vi "Main.vi"(11 "Module Admin":refnum<class "Delacor_lib_QMH_Module Admin.lvclass">) -> ()   [LabVIEW 2019, in "Analysis.lvlib"]
doc: "This template is based off of the Queued Message Handler design pattern and the Queued Message Handler project template that ships with LabVIEW.\n\nThe main difference is that the queue is private to this module and communication between modules is performed via Broadcast and Request events.\n\nRequest events are wrapped in public API methods and are handled in the Event Handling Loop (EHL) of this VI. Any module can register for Broadcast events sent by this module. The EHL generates messages based on user interface actions.\n\nThe Message Handling Loop (MHL) processes messages generated by the EHL, or by other messages. The messages are string values, so new messages can be added easily to the Message Cases case structure in the MHL. Each message cluster can also provide an optional value for Message Data, which is a variant that can be converted to whatever message-specific data is required.\n_____\nBased on Delacor QMH Project Template 4.0.0.47.\n_____\nBased on DQMH Project Template 6.1.0.94."
uses:
  Analysis.lvlib
  <vilib>/Delacor/Delacor QMH/Libraries/Module Admin_class/Delacor_lib_QMH_Module Admin.lvclass
  Module Data--cluster.ctl
  Neo-Laura-LVOOP/Class Library/Fcurve_class/Fcurve.lvclass
  Main UI Shared/Decimation input --cluster.ctl
  Stop Argument--cluster.ctl
  <vilib>/Delacor/Delacor QMH/Libraries/Message Queue_class/Delacor_lib_QMH_Message Queue.lvclass/Delacor_lib_QMH_Message Queue.ctl
  <vilib>/Delacor/Delacor QMH/Libraries/Module Admin_class/Delacor_lib_QMH_Module Admin.lvclass/Delacor_lib_QMH_Module Admin.ctl
  Update analysis parameters Argument--cluster.ctl
  Update analysis parameters (Reply Payload)--cluster.ctl
  Update Savitzky parameters Argument--cluster.ctl
  Update decimation Argument--cluster.ctl
  Update contact parameters Argument--cluster.ctl
  Update Tau delay (ms) Argument--cluster.ctl
  Open Fcurve object Argument--cluster.ctl
  Neo-Laura-LVOOP/SignalViewer/TDMS_DataHandler_class/Fcurve Meta data.ctl
  Open Fcurve object (Reply Payload)--cluster.ctl
  Neo-Laura-LVOOP/Class Library/Fcurve_class/Metadata.ctl
  <vilib>/Utility/miscctls.llb/LVPointTypeDef.ctl
  <vilib>/Delacor/Delacor QMH/Libraries/Message Queue_class/Delacor_lib_QMH_Enqueue Message (Single).vi
  <vilib>/Delacor/Delacor QMH/Libraries/Module Admin_class/Delacor_lib_QMH_Get External Launch.vi
  <vilib>/Utility/error.llb/Error Cluster From Error Code.vi
  <vilib>/ErrorRing/Error Ring.xnode
  <vilib>/Delacor/Delacor QMH/Libraries/Message Queue_class/Delacor_lib_QMH_Message Queue.lvclass
  Settings Editor/Settings Editor.lvlib
  Main UI Shared/MAIN UI Shared.lvlib
  Neo-Laura-LVOOP/SignalViewer/TDMS_DataHandler_class/TDMS_DataHandler.lvclass
panel:
  out "Settings":T1={"Contact"={"Contact stat?"=TRUE, "Contact Spread of dev"=0.0}, "Decimation"={"App"={"Dec"=1, "apply"=FALSE}, "Con"={"Dec"=1, "apply"=FALSE}, "Ret"={"Dec"=1, "apply"=FALSE}}, "Savitzksky-Golay"={"Sidepoints (M)"=20.0, "Filter Order"=5}, "Fcurve Metadata"=[], "Tau Delay (ms)"=0.0, "Fcurve obj"=refnum} {"Savitzksky-Golay"."Filter Order" scale=0.0..10.0; "Savitzksky-Golay"."Sidepoints (M)" scale=0.0..10.0; "Contact"."Contact Spread of dev" format="%#_13g"}
  out "error out":errorcluster
  # "This is a headless module. Show its panel to confirm that the Settings are updated correctly and other debugging tasks. Use the Settings Editor to change the settings for this module."
  # "Contact"
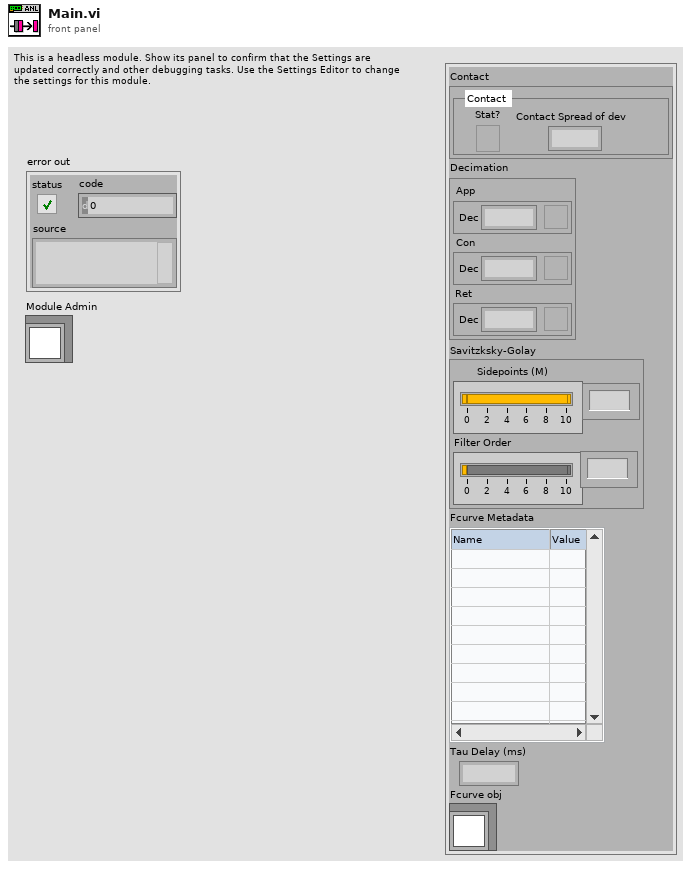
[diagram p1: front panel]
types:
  T1 = typedef "Analysis.lvlib/Module Data--cluster.ctl" = cluster{"Contact":cluster{"Contact stat?":bool, "Contact Spread of dev":dbl}, "Decimation":T2, "Savitzksky-Golay":cluster{"Sidepoints (M)":dbl, "Filter Order":i32}, "Fcurve Metadata":string[][], "Tau Delay (ms)":dbl, "Fcurve obj":refnum<class "Fcurve.lvclass">}
  T2 = typedef "MAIN UI Shared.lvlib/Decimation input --cluster.ctl" = cluster{"App":cluster{"Dec":i32, "apply":bool}, "Con":cluster{"Dec":i32, "apply":bool}, "Ret":cluster{"Dec":i32, "apply":bool}}
  T3 = typedef "Settings Editor.lvlib/Broadcast Events--cluster.ctl" = cluster{"Module Did Init":refnum<user-event>, "Status Updated":refnum<user-event>, "Error Reported":refnum<user-event>, "Module Did Stop":refnum<user-event>, "Update Module Execution Status":refnum<user-event>, "TDMS path settings updated":refnum<user-event>}
  T4 = typedef "Analysis.lvlib/Request Events--cluster.ctl" = cluster{"Stop Module":refnum<user-event>, "Show Panel":refnum<user-event>, "Hide Panel":refnum<user-event>, "Get Module Execution Status":refnum<user-event>, "Show Diagram":refnum<user-event>, "Wakeup Helper Loop":refnum<user-event>, "Change Settings":refnum<user-event>, "Update analysis parameters":refnum<user-event>, "Update Savitzky parameters":refnum<user-event>, "Update decimation":refnum<user-event>, "Update contact parameters":refnum<user-event>, "Update Tau delay (ms)":refnum<user-event>, "Open Fcurve object":refnum<user-event>}
  T5 = enum32{"invalid lock state", "Not Locked", "Locked (No Password)", "Password-protected"}
  T6 = typedef "Analysis.lvlib/Stop Argument--cluster.ctl" = cluster{"Origin":string, "Exit via Stop Module Req?":bool, "Wait for Module to stop?":bool}
  T7 = typedef "Analysis.lvlib/Update analysis parameters Argument--cluster.ctl" = cluster{"Contact":cluster{"Contact stat?":bool, "Contact Spread of dev":dbl}, "Decimation":T2, "Savitzksky-Golay":cluster{"Sidepoints (M)":dbl, "Filter Order":i32}, "Wait Notifier":refnum<notifier>, "wait for reply":bool}
  T8 = typedef "Analysis.lvlib/Update Savitzky parameters Argument--cluster.ctl" = cluster{"Savitzksky-Golay":cluster{"Sidepoints (M)":dbl, "Filter Order":i32}}
  T9 = typedef "Analysis.lvlib/Update decimation Argument--cluster.ctl" = cluster{"Decimation":T2}
  T10 = typedef "Analysis.lvlib/Update contact parameters Argument--cluster.ctl" = cluster{"Contact":cluster{"Contact stat?":bool, "Contact Spread of dev":dbl}}
  T11 = typedef "Analysis.lvlib/Update Tau delay (ms) Argument--cluster.ctl" = cluster{"Tau Delay (ms)":dbl}
  T12 = typedef "Analysis.lvlib/Open Fcurve object Argument--cluster.ctl" = cluster{"Group metadata":T13, "Channel name(s)":string[], "Channel datum out":waveform(dbl)[], "Wait Notifier":refnum<notifier>, "wait for reply":bool}
  T13 = typedef "TDMS_DataHandler.lvclass/Fcurve Meta data.ctl" = cluster{"property names":string[], "property values":variant[]}
  T14 = typedef "LVPointTypeDef.ctl" = cluster{"Horizontal":i16, "Vertical":i16}
  T15 = enum32{"Invalid", "Standard", "Closed", "Hidden", "Minimized", "Maximized"}
  T16 = typedef "Analysis.lvlib/Update analysis parameters (Reply Payload)--cluster.ctl" = cluster{"updated":bool, "error":errorcluster}
  T17 = typedef "Analysis.lvlib/Open Fcurve object (Reply Payload)--cluster.ctl" = cluster{"Fcurve out":cluster{"X":dbl[], "Y":dbl[]}[], "Metadata out":T18, "error":errorcluster}
  T18 = typedef "Fcurve.lvclass/Metadata.ctl" = cluster{"dt (us)":dbl, "Dec Factor":dbl, "Z piezo Sensitivity (nm/V)":dbl, "K (N/m)":dbl, "Sp (V)":dbl, "Contact (ms)":dbl, "Zpos contact":dbl, "Vel_app (nm/s)":dbl, "Vel_ret (nm/s)":dbl, "deltaV (nm)":dbl, "Def_V0 (v)":dbl, "Piezo gain":dbl, "invOLS (nm/V)":dbl}
  T19 = cluster{"Contact stat?":bool, "Contact Spread of dev":dbl}
  T20 = cluster{"Sidepoints (M)":dbl, "Filter Order":i32}
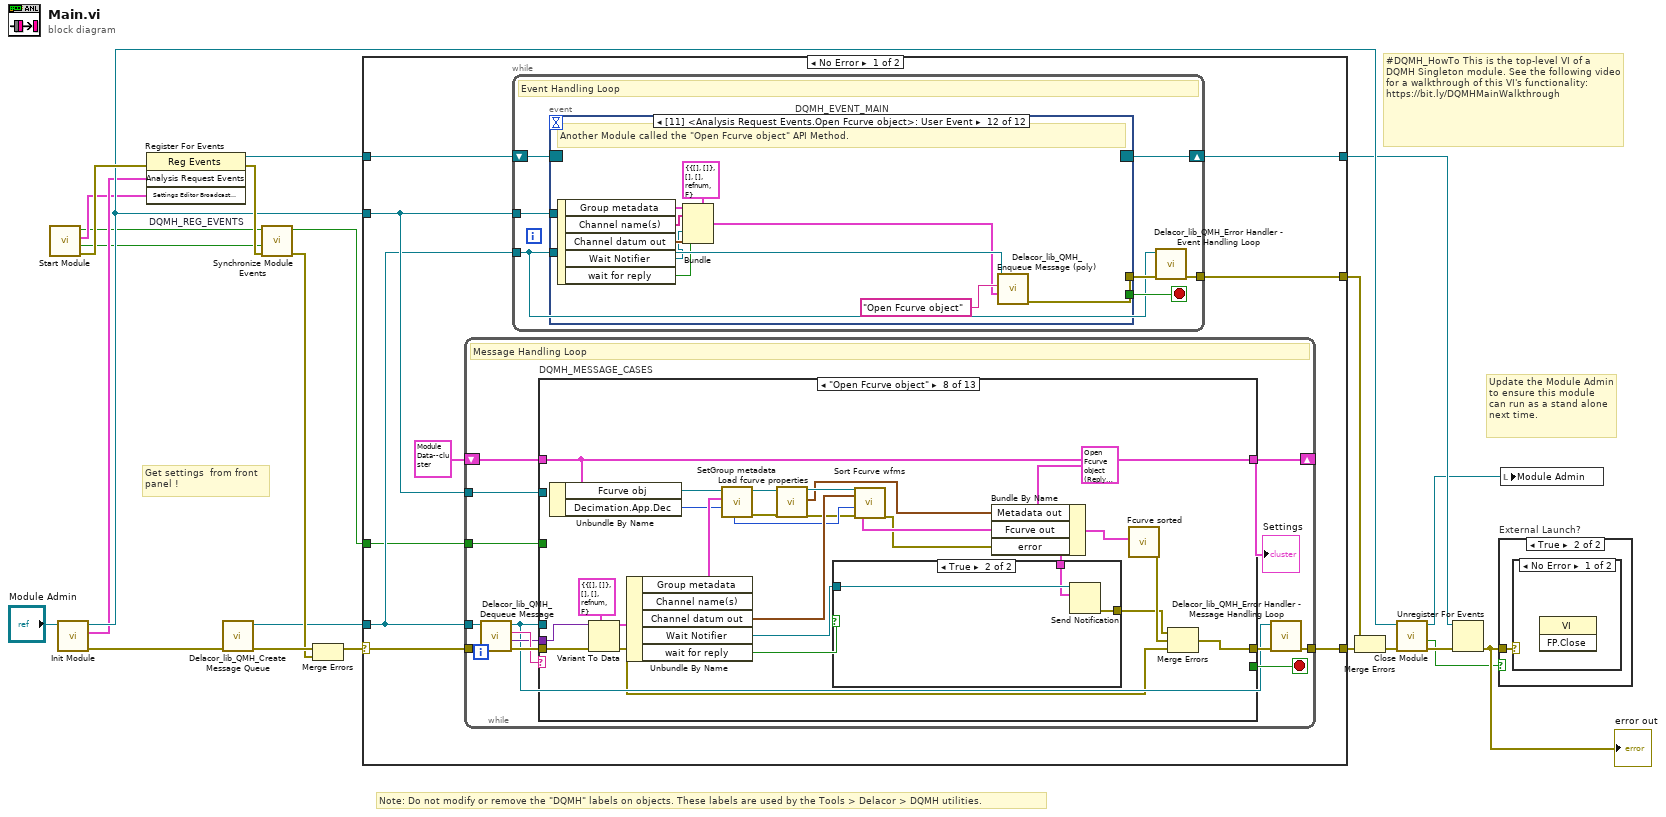
[diagram p0: block diagram]
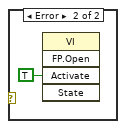
[diagram p3: hidden frame]
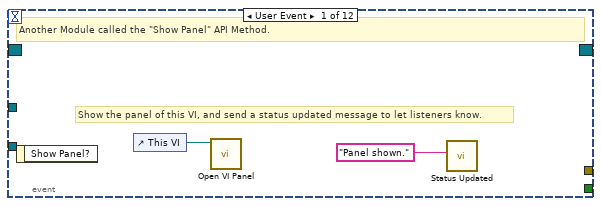
[diagram p4: hidden frame]
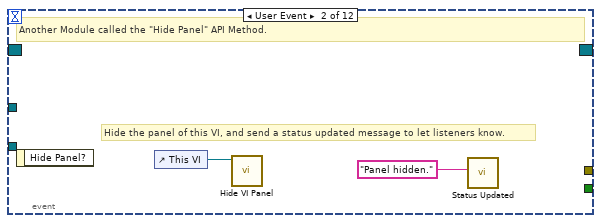
[diagram p5: hidden frame]
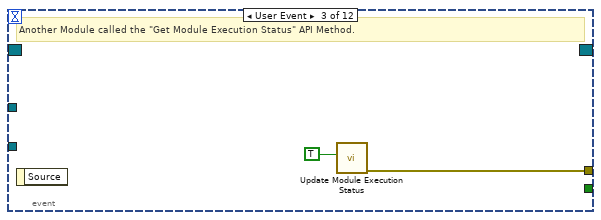
[diagram p6: hidden frame]
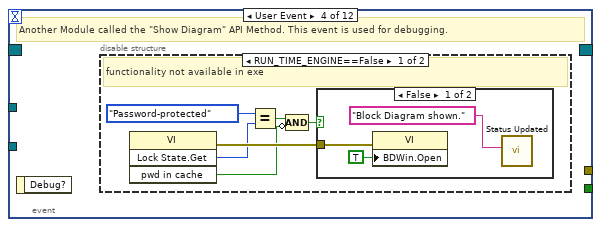
[diagram p7: hidden frame]
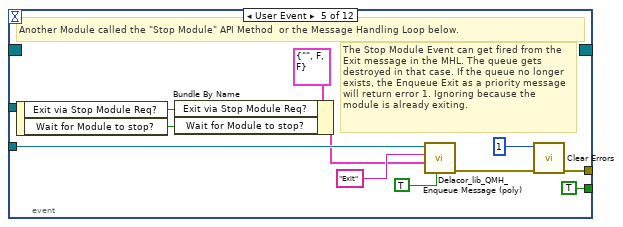
[diagram p10: hidden frame]
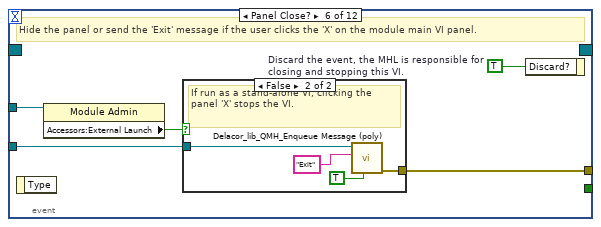
[diagram p11: hidden frame]
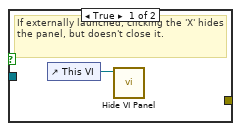
[diagram p12: hidden frame]
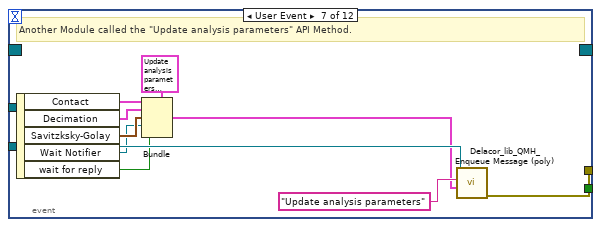
[diagram p13: hidden frame]
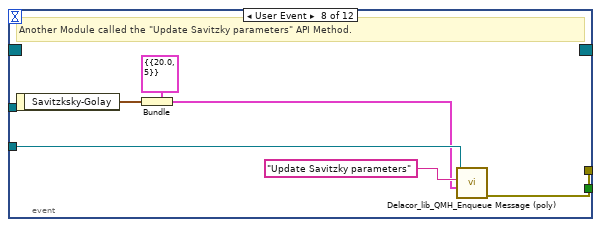
[diagram p14: hidden frame]
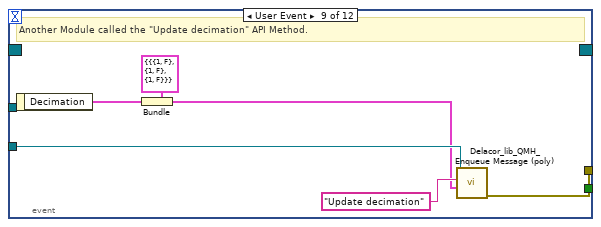
[diagram p15: hidden frame]
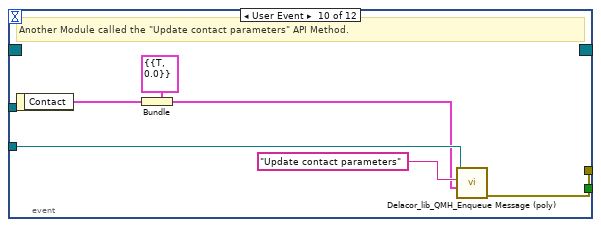
[diagram p16: hidden frame]
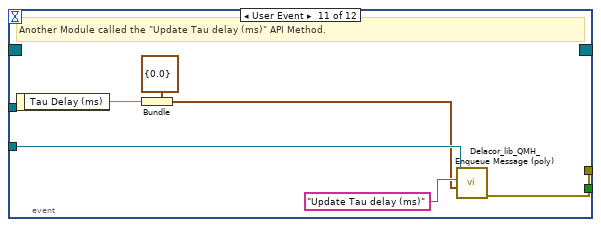
[diagram p17: hidden frame]
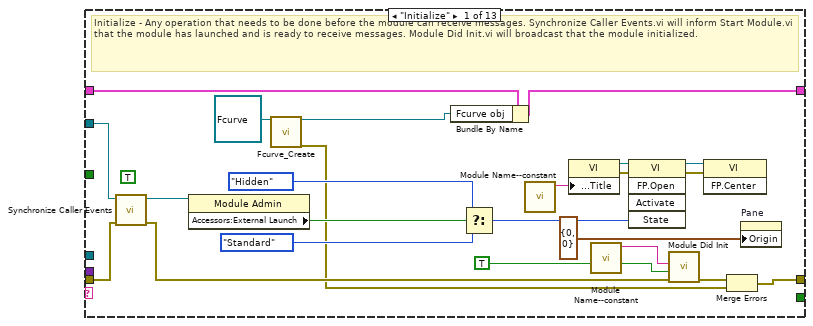
[diagram p18: hidden frame]
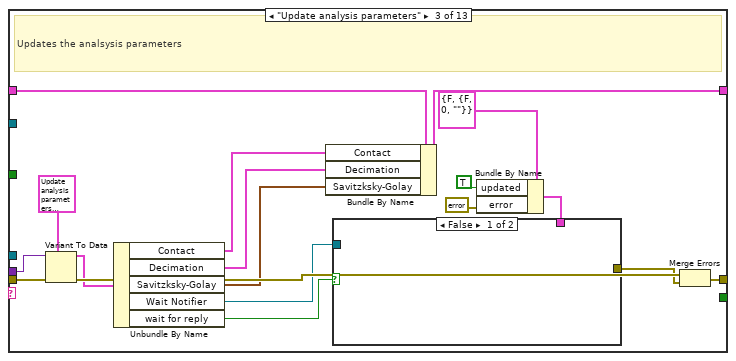
[diagram p20: hidden frame]
diagram:
  # "Get settings  from front\npanel !"
  # "#DQMH_HowTo This is the top-level VI of a DQMH Singleton module. See the following video for a walkthrough of this VI's functionality: https://bit.ly/DQMHMainWalkthrough"
  # "Note: Do not modify or remove the \"DQMH\" labels on objects. These labels are used by the Tools > Delacor > DQMH utilities."
  # "Update the Module Admin to ensure this module can run as a stand alone next time."
  n1 = call "Start Module.vi"() -> ("error out"=w15:errorcluster, "Wait for Event Sync?"=w2:bool, "Settings Editor Broadcast Events"=w3:T3, "Module Was Already Running?"=w1:bool)  [unwired: 8 in]
  n2 = call "Init Module.vi"("Singleton Module Admin in"="Module Admin") -> ("error out"=w21:errorcluster, "Analysis Request Events"=w4:T4, "Singleton Module Admin out"=w11:refnum<class "Delacor_lib_QMH_Module Admin.lvclass">)  [unwired: 8 in]
  n3 = register-events "DQMH_REG_EVENTS"(error in=w15, w4, w3) -> (reference out=w9:refnum<event-registration>, error out=w14:errorcluster)  [unwired: 1 in]
  n4 = call <vilib>:"Delacor_lib_QMH_Create Message Queue.vi"("error in"=w21) -> ("error out"=w17:errorcluster, "Message Queue"=w8:refnum<class "Delacor_lib_QMH_Message Queue.lvclass">)  [unwired: 9 in]
  n5 = call "Synchronize Module Events.vi"("error in (no error)"=w14, "Wait for Event Sync?"=w2) -> ("error out"=w13:errorcluster)  [unwired: 9 in]
  n6 = Merge Errors(w17, w13) -> (w16:errorcluster)
  n7 = case shown="No Error" w16 {
    selector: w16 -> [w29 w303]
    tunnel: [w31 w302] -> w22
    tunnel: [w28 w310] -> w10
    tunnel: w9 -> [w27 w310]
    tunnel: w8 -> [w25 w304]
    tunnel: [w30 _] -> w20
    tunnel: w11 -> [w26 w306]
    tunnel: w1 -> [w23 w305]
    frame No Error {
      n8 = while {
        tunnel: w25 -> [w122]
        shift-right: [w126] -> _
        shift-left: T1 {"Contact"={"Contact stat?"=TRUE, "Contact Spread of dev"=0.0}, "Decimation"={"App"={"Dec"=1, "apply"=FALSE}, "Con"={"Dec"=1, "apply"=FALSE}, "Ret"={"Dec"=1, "apply"=FALSE}}, "Savitzksky-Golay"={"Sidepoints (M)"=20.0, "Filter Order"=5}, "Fcurve Metadata"=[[""]], "Tau Delay (ms)"=0.0, "Fcurve obj"=refnum} ("Data Cluster") -> [w127]
        tunnel: w29 -> [w130]
        tunnel: [w128] -> w31
        tunnel: w26 -> [w120]
        tunnel: w23 -> [w119]
        stop <- w125 stop-if-true
        # "Message Handling Loop"
        n9 = call-dynamic "Delacor_lib_QMH_Dequeue Message.vi"("error in"=w130, "Message Queue in"=w122) -> ("error out"=w129:errorcluster, "Message Data"=w123:variant, "Message"=w124:string, "Message Queue out"=w121:refnum<class "Delacor_lib_QMH_Message Queue.lvclass">)  [unwired: 6 in]
        n10 = case "DQMH_MESSAGE_CASES" shown="\"Open Fcurve object\"" w124 {
          selector: w124 -> [_ _ _ _ _ _ _ _ _ _ _ _ w289]
          tunnel: w121 -> [_ _ _ _ _ _ _ _ _ _ w254 w279 _]
          tunnel: w129 -> [w152 w156 w174 w185 w193 w198 w219 w243 w249 w251 w261 w285 w292]
          tunnel: [w149 w156 w165 w184 w192 w197 w218 w234 w248 w251 w257 w282 w293] -> w131
          tunnel: w127 -> [w134 w155 w164 w180 w188 w195 w214 w231 w247 w250 w256 w270 w290]
          tunnel: [w133 w155 w163 w179 w187 w194 w213 w231 w247 w250 w256 w270 w290] -> w126
          tunnel: [_ _ _ _ _ _ _ _ _ _ _ w278 _] -> w125
          tunnel: w123 -> [_ _ w172 w183 w191 w196 w217 w241 _ _ w255 w277 _]
          tunnel: w120 -> [w141 _ _ _ _ _ _ _ _ _ w253 w272 _]
          tunnel: w119 -> [_ _ _ _ _ _ _ _ _ _ _ w271 _]
          frame "Initialize" {
            (unwired) TRUE ("wait for reply (T)")
            # "Initialize - Any operation that needs to be done before the module can receive messages. Synchronize Caller Events.vi will inform Start Module.vi that the module has launched and is ready to receive messages. Module Did Init.vi will broadcast that the module initialized."
            n11 = call "Synchronize Caller Events.vi"("error in (no error)"=w152, "Singleton Module Admin in"=w141) -> ("error out"=w151:errorcluster, "Singleton Module Admin out"=w138:refnum<class "Delacor_lib_QMH_Module Admin.lvclass">)  [unwired: 8 in]
            n12 = property class="Module Admin"(reference=w138) -> ("Accessors:External Launch"=w145:bool)  [unwired: 1 in, 2 out]
            n13 = call "Fcurve_Create.vi"("reference in"=refnum<class "Fcurve.lvclass"> refnum) -> ("reference out"=w132:refnum<class "Fcurve.lvclass">, "error out"=w135:errorcluster)  [unwired: 17 in]
            n14 = Bundle By Name(cluster=w134, "Fcurve obj"=w132) -> (w133:T1)
            n15 = Select(t=T15."Hidden" ("State"), s=w145, f=T15."Standard" ("State")) -> (s? t:f=w142:T15)
            n16 = call "Module Name--constant.vi"() -> ("Module Name"=w148:string)  [unwired: 11 in]
            n17 = property class="VI"("Front Panel.Title"=w148) -> (reference out=w147:refnum<vi>, error out=w154:errorcluster)  [unwired: 2 in]
            n18 = call "Module Name--constant.vi"() -> ("Module Name"=w139:string)  [unwired: 11 in]
            n19 = invoke class="VI" method="FP.Open"(reference=w147, error in=w154, "State"=w142) -> (reference out=w146:refnum<vi>, error out=w153:errorcluster)  [unwired: 2 in, 3 out]
            n20 = call "Module Did Init.vi"("error in (no error)"=w151, "Initialized?"=TRUE, "Origin"=w139) -> ("error out"=w150:errorcluster)  [unwired: 8 in]
            n21 = invoke class="VI" method="FP.Center"(reference=w146, error in=w153) -> ()  [unwired: 1 in, 3 out]
            n22 = Merge Errors(w150, w135) -> (w149:errorcluster)
            n23 = property on="Pane" class="Pane"("Origin"=T14 {"Horizontal"=0, "Vertical"=0}) -> ()  [unwired: 2 in, 2 out]
          }
          frame "---Module Specific---" {
            # "Separator -- The following cases handle messages specific to this Module."
          }
          frame "Update analysis parameters" {
            # "Updates the analsysis parameters"
            n24 = Variant To Data(error in=w174, type=T7 {"Contact"={"Contact stat?"=TRUE, "Contact Spread of dev"=0.0}, "Decimation"={"App"={"Dec"=1, "apply"=FALSE}, "Con"={"Dec"=1, "apply"=FALSE}, "Ret"={"Dec"=1, "apply"=FALSE}}, "Savitzksky-Golay"={"Sidepoints (M)"=20.0, "Filter Order"=5}, "Wait Notifier"=refnum, "wait for reply"=FALSE} ("Update analysis parameters Argument"), Variant=w172) -> (data=w170:T7, error out=w173:errorcluster)
            n25 = Unbundle By Name(w170) -> ("Contact"=w162:T19, "Decimation"=w161:T2, "Savitzksky-Golay"=w160:T20, "Wait Notifier"=w169:refnum<notifier>, "wait for reply"=w168:bool)
            n26 = Bundle By Name(cluster=w164, "Contact"=w162, "Decimation"=w161, "Savitzksky-Golay"=w160) -> (w163:T1)
            n27 = Bundle By Name(cluster=T16 {"updated"=FALSE, "error"={"status"=FALSE, "code"=0, "source"=""}} ("Update analysis parameters (Reply Payload)"), "updated"=TRUE, "error"=errorcluster {"status"=FALSE, "code"=0, "source"=""}) -> (w167:T16)
            n28 = case shown="False" w168 {
              tunnel: w169 -> [_ w177]
              tunnel: w167 -> [_ w176]
              tunnel: [_ w175] -> w158
              frame False {
              }
              frame True {
                n29 = Send Notification(notification=w176, notifier=w177) -> (error out=w175:errorcluster)  [unwired: 1 in, 1 out]
              }
            }
            n30 = Merge Errors(w173, w158) -> (w165:errorcluster)
          }
          frame "Update Savitzky parameters" {
            # "Updates savistky parmeters on analysis module"
            n31 = Variant To Data(error in=w185, type=T8 {"Savitzksky-Golay"={"Sidepoints (M)"=20.0, "Filter Order"=5}} ("Update Savitzky parameters Argument"), Variant=w183) -> (data=w181:T8, error out=w184:errorcluster)
            n32 = Unbundle By Name(w181) -> ("Savitzksky-Golay"=w178:T20)
            n33 = Bundle By Name(cluster=w180, "Savitzksky-Golay"=w178) -> (w179:T1)
          }
          frame "Update decimation" {
            # "Updates decimation value"
            n34 = Variant To Data(error in=w193, type=T9 {"Decimation"={"App"={"Dec"=1, "apply"=FALSE}, "Con"={"Dec"=1, "apply"=FALSE}, "Ret"={"Dec"=1, "apply"=FALSE}}} ("Update decimation Argument"), Variant=w191) -> (data=w189:T9, error out=w192:errorcluster)
            n35 = Unbundle By Name(w189) -> ("Decimation"=w186:T2)
            n36 = Bundle By Name(cluster=w188, "Decimation"=w186) -> (w187:T1)
          }
          frame "Update contact parameters" {
            # "Updates contact parmaeters from main gui"
            n37 = in-place {
              in-place-border: w198 -> [w211]
              in-place-border: [w203] -> w197
              in-place-border: w196 -> [w210]
              n38 = in-place-cluster #1(w195) -> ("Fcurve obj"=w206:refnum<class "Fcurve.lvclass">)  [unwired: 1 out]
              n39 = Variant To Data(error in=w211, type=T10 {"Contact"={"Contact stat?"=TRUE, "Contact Spread of dev"=0.0}} ("Update contact parameters Argument"), Variant=w210) -> (data=w208:T10, error out=w204:errorcluster)
              n40 = Unbundle By Name(w208) -> ("Contact"=w201:T19, "Contact.Contact stat?"=w200:bool, "Contact.Contact Spread of dev"=w199:dbl)
              n41 = call-dynamic "SetContact stat.vi"("error in (no error)"=w204, "Contact stat"=w200, "reference in"=w206) -> ("error out"=w202:errorcluster, "reference out"=w207:refnum<class "Fcurve.lvclass">)  [unwired: 7 in]
              n42 = call-dynamic "SetContact Spread of dev.vi"("error in (no error)"=w202, "Contact Spread of dev"=w199, "reference in"=w207) -> ("error out"=w203:errorcluster, "reference out"=w205:refnum<class "Fcurve.lvclass">)  [unwired: 7 in]
              n43 = in-place-cluster #1("Contact"=w201, "Fcurve obj"=w205) -> (w194:T1)
            }
          }
          frame "Update Tau delay (ms)" {
            # "Updates tau delay (ms)"
            n44 = Variant To Data(error in=w219, type=T11 {"Tau Delay (ms)"=0.0} ("Update Tau delay (ms) Argument"), Variant=w217) -> (data=w215:T11, error out=w218:errorcluster)
            n45 = Unbundle By Name(w215) -> ("Tau Delay (ms)"=w212:dbl)
            n46 = Bundle By Name(cluster=w214, "Tau Delay (ms)"=w212) -> (w213:T1)
          }
          frame "Open Fcurve object" {
            n47 = Unbundle By Name(w231) -> ("Fcurve obj"=w229:refnum<class "Fcurve.lvclass">, "Decimation.App.Dec"=w227:i32)
            n48 = Variant To Data(error in=w243, type=T12 {"Group metadata"={"property names"=[], "property values"=[]}, "Channel name(s)"=[], "Channel datum out"=[], "Wait Notifier"=refnum, "wait for reply"=FALSE} ("Open Fcurve object Argument"), Variant=w241) -> (data=w239:T12, error out=w242:errorcluster)
            n49 = Unbundle By Name(w239) -> ("Group metadata"=w230:T13, "Channel datum out"=w228:waveform(dbl)[], "Wait Notifier"=w238:refnum<notifier>, "wait for reply"=w237:bool)  [unwired: 1 out]
            n50 = call-dynamic "SetGroup metadata.vi"("Group metadata"=w230, "reference in"=w229) -> ("error out"=w222:errorcluster, "reference out"=w224:refnum<class "Fcurve.lvclass">)  [unwired: 8 in]
            n51 = call-dynamic "Load fcurve properties.vi"("reference in"=w224, "error in (no error)"=w222) -> ("reference out"=w223:refnum<class "Fcurve.lvclass">, "Metadata out"=w220:T18, "error out"=w221:errorcluster)  [unwired: 15 in]
            n52 = call-dynamic "Sort Fcurve wfms.vi"("reference in"=w223, "Channels In"=w228, "decimating factor"=w227, "error in (no error)"=w221) -> ("Fcurve out"=w226:cluster{"X":dbl[], "Y":dbl[]}[], "error out"=w225:errorcluster)  [unwired: 10 in, 4 out]
            n53 = Bundle By Name(cluster=T17 {"Fcurve out"=[], "Metadata out"={"dt (us)"=2.0, "Dec Factor"=1.0, "Z piezo Sensitivity (nm/V)"=6000.0, "K (N/m)"=0.6, "Sp (V)"=16.0, "Contact (ms)"=0.0, "Zpos contact"=2.000001, "Vel_app (nm/s)"=10000.0, "Vel_ret (nm/s)"=100000.0, "deltaV (nm)"=600.0, "Def_V0 (v)"=-0.113287, "Piezo gain"=1.0, "invOLS (nm/V)"=23.8}, "error"={"status"=FALSE, "code"=0, "source"=""}} ("Open Fcurve object (Reply Payload)"), "Metadata out"=w220, "Fcurve out"=w226, "error"=w225) -> (w236:T17)
            n54 = case shown="True" w237 {
              tunnel: w238 -> [_ w246]
              tunnel: w236 -> [_ w245]
              tunnel: [_ w244] -> w232
              frame False {
              }
              frame True {
                n55 = Send Notification(notification=w245, notifier=w246) -> (error out=w244:errorcluster)  [unwired: 1 in, 1 out]
              }
            }
            n56 = call "Fcurve sorted.vi"("Reply Payload"=w236) -> ("error out"=w233:errorcluster)  [unwired: 10 in]
            n57 = Merge Errors(w232, w233, w242) -> (w234:errorcluster)
          }
          frame "---Copy This Frame---" {
            # "Duplicate this frame when creating new messages.  Change this comment in the duplicated frame to describe this message."
            n58 = Merge Errors(w249) -> (w248:errorcluster)
          }
          frame "---Exit and Error Handling---" {
            # "Separator - The following cases handle errors and exit messages."
          }
          frame "Error" {
            # "Error - Check the error message data and respond accordingly. This message is sent by the \"Error Handler\" VIs at the end of each loop in this application."
            n59 = property class="Module Admin"(reference=w253) -> ("Accessors:External Launch"=w252:bool)  [unwired: 1 in, 2 out]
            n60 = Variant To Data(error in=w261, type=errorcluster {"status"=FALSE, "code"=0, "source"=""} ("error constant"), Variant=w255) -> (data=w262:errorcluster, error out=w259:errorcluster)
            n61 = call "Error Reported.vi"("Error"=w262) -> ()  [unwired: 10 in, 1 out]
            n62 = case shown="False" w252 {
              tunnel: [w267 _] -> w258
              tunnel: w254 -> [w265 _]
              tunnel: w262 -> [w266 _]
              frame False {
                # "If the module is running standalone, then pop up an error dialog and call the \"Exit\" message."
                n63 = call <vilib>:"Simple Error Handler.vi"("error in (no error)"=w266) -> ()  [unwired: 4 in, 5 out]
                n64 = call-poly <vilib>:"Delacor_lib_QMH_Enqueue Message (poly).vi"("Priority Message? (F)"=TRUE, "Message"="Exit", "Message Queue in"=w265) -> ("error out"=w267:errorcluster)  [unwired: 7 in, 1 out]
              }
              frame True {
                # "If the module was launched externally, calling the Error Reported broadcast VI is the only action performed by the \"Error\" message. The module's caller can then process the error appropriately."
              }
            }
            n65 = Merge Errors(w259, w258) -> (w257:errorcluster)
            n66 = local write "error out"(w257) -> ()
          }
          frame "Exit" {
            w276 = 91  # 91: not all Exit messages will have an argument
            w278 = TRUE  # Stop the VI
            # "Release the message queue reference"
            # "Exit - Exit the application."
            n67 = Variant To Data(error in=w285, type=T6 {"Origin"="", "Exit via Stop Module Req?"=FALSE, "Wait for Module to stop?"=FALSE} ("Stop Argument"), Variant=w277) -> (data=w274:T6, error out=w281:errorcluster)
            n68 = call <vilib>:"Clear Errors.vi"("error in (no error)"=w281, "specific error code to clear (0: all)"=w276) -> ("error out"=w284:errorcluster)  [unwired: 4 in, 1 out]
            n69 = Unbundle By Name(w270) -> ("Fcurve obj"=w269:refnum<class "Fcurve.lvclass">)
            n70 = call-dynamic "Destroy.vi"("reference in"=w269) -> ("error out"=w268:errorcluster)  [unwired: 17 in, 1 out]
            n71 = control-ref of="This VI"() -> (w273:refnum<vi>)
            n72 = call "Handle Exit.vi"("Stop Argument"=w274, "Admin in"=w272, "VI reference"=w273) -> ("error out"=w280:errorcluster)  [unwired: 7 in, 1 out]
            n73 = call-dynamic "Delacor_lib_QMH_Release Message Queue.vi"("error in"=w284, "Message Queue"=w279) -> ("error out"=w283:errorcluster)  [unwired: 9 in]
            n74 = case "Settings Editor was\nalready running?" shown="False" w271 {
              frame False {
                n75 = call "Module Name--constant.vi"() -> ("Module Name"=w287:string)  [unwired: 11 in]
                n76 = call "Stop Module.vi"("Wait for Module to Stop? (F)"=TRUE, "Origin"=w287) -> ()  [unwired: 9 in, 1 out]
              }
              frame True {
                # "Another Module is\nin charge of stopping Settings Editor"
              }
            }
            n77 = Merge Errors(w268, w283, w280) -> (w282:errorcluster)
          }
          frame Default {
            # "'Default' case only runs if there is a message that isn't defined in any of the other cases.  Output a programming error."
            n78 = call "Module Name--constant.vi"() -> ("Module Name"=w288:string)  [unwired: 11 in]
            n79 = xnode "Error Ring"("parameter 0"=w289, "parameter 1"=w288) -> ("error out"=w291:errorcluster)
            n80 = Merge Errors(w292, w291) -> (w293:errorcluster)
          }
        }
        "Settings" <- w126
        n81 = call-dynamic "Delacor_lib_QMH_Error Handler - Message Handling Loop.vi"("error in"=w131, "Message Queue in"=w121) -> ("dup error in"=w128:errorcluster)  [unwired: 8 in, 1 out]
      }
      n82 = while {
        tunnel: w25 -> [w32]
        shift-right: [w35] -> w28
        shift-left: w27 -> [w36]
        tunnel: [w37] -> w30
        tunnel: w26 -> [w33]
        stop <- w34 stop-if-true
        # "Event Handling Loop"
        n83 = event "DQMH_EVENT_MAIN" shown="[11] <Analysis Request Events.Open Fcurve object>: User Event" {
          selector: w36 -> [_ _ _ _ _ _ _ _ _ _ _ _]
          dyn-events: [_ _ _ _ _ _ _ _ _ _ _ _] -> w35
          timeout: _ -> [_ _ _ _ _ _ _ _ _ _ _ _]
          tunnel: [_ _ _ _ TRUE ("Discard?") _ _ _ _ _ _ _] -> w34
          tunnel: w32 -> [_ _ _ _ w60 w67 w84 w90 w96 w102 w108 w118]
          tunnel: [_ _ w44 _ w63 w69 w75 w85 w91 w97 w103 w109] -> w38
          tunnel: w33 -> [_ _ _ _ _ w66 _ _ _ _ _ _]
          event User Event {
            # "Show the panel of this VI, and send a status updated message to let listeners know."
            # "Another Module called the \"Show Panel\" API Method."
            n84 = event-data() -> ()  [unwired: 1 in, 1 out]
            n85 = control-ref of="This VI"() -> (w40:refnum<vi>)
            n86 = call "Open VI Panel.vi"("VI"=w40) -> ()  [unwired: 10 in, 1 out]
            n87 = call "Status Updated.vi"("Status"="Panel shown." ("format string")) -> ()  [unwired: 10 in, 1 out]
          }
          event User Event {
            # "Hide the panel of this VI, and send a status updated message to let listeners know."
            # "Another Module called the \"Hide Panel\" API Method."
            n88 = event-data() -> ()  [unwired: 1 in, 1 out]
            n89 = control-ref of="This VI"() -> (w42:refnum<vi>)
            n90 = call "Hide VI Panel.vi"("VI"=w42) -> ()  [unwired: 10 in, 1 out]
            n91 = call "Status Updated.vi"("Status"="Panel hidden." ("format string")) -> ()  [unwired: 10 in, 1 out]
          }
          event User Event {
            # "Another Module called the \"Get Module Execution Status\" API Method."
            n92 = event-data() -> ()  [unwired: 1 in, 1 out]
            n93 = call "Update Module Execution Status.vi"("Running?"=TRUE) -> ("error out"=w44:errorcluster)  [unwired: 10 in]
          }
          event User Event {
            # "Another Module called the \"Show Diagram\" API Method. This event is used for debugging."
            n94 = event-data() -> ()  [unwired: 1 in, 1 out]
            n95 = disable-structure shown="RUN_TIME_ENGINE==False" {
              frame condition #0 (active) {
                # "functionality not available in exe"
                n96 = invoke class="VI" method="Lock State.Get"() -> (error out=w50:errorcluster, "Get Lock State"=w49:T5, "pwd in cache"=w46:bool)  [unwired: 4 in, 1 out]
                n97 = Equal?(x=T5."Password-protected", y=w49) -> (x = y?=w47:bool)
                n98 = Compound Arithmetic op=AND(w47, invert w46) -> (w45:bool)
                n99 = case shown="False" w45 {
                  tunnel: w50 -> [w53 _]
                  frame False {
                    n100 = property class="VI"(error in=w53, "BDWin.Open"=TRUE ("Block Diagram Window:Open")) -> ()  [unwired: 1 in, 2 out]
                    n101 = call "Status Updated.vi"("Status"="Block Diagram shown." ("format string")) -> ()  [unwired: 10 in, 1 out]
                  }
                  frame True {
                    # "Password-protected VI, and the password is not in the cache. Do not show the diagram."
                  }
                }
              }
              frame condition #1 {
              }
            }
          }
          event User Event {
            # "The Stop Module Event can get fired from the Exit message in the MHL. The queue gets destroyed in that case. If the queue no longer exists, the Enqueue Exit as a priority message will return error 1. Ignoring because the module is already exiting."
            # "Another Module called the \"Stop Module\" API Method  or the Message Handling Loop below."
            n102 = event-data() -> ("Exit via Stop Module Req?"=w56:bool, "Wait for Module to stop?"=w55:bool)  [unwired: 1 in]
            n103 = Bundle By Name(cluster=T6 {"Origin"="", "Exit via Stop Module Req?"=FALSE, "Wait for Module to stop?"=FALSE} ("Stop Argument"), "Exit via Stop Module Req?"=w56, "Wait for Module to stop?"=w55) -> (w54:T6)
            n104 = call-poly <vilib>:"Delacor_lib_QMH_Enqueue Message (poly).vi"("Priority Message? (F)"=TRUE, "Message Data"=w54, "Message"="Exit", "Message Queue in"=w60) -> ("error out"=w64:errorcluster)  [unwired: 6 in, 1 out]
            n105 = call <vilib>:"Clear Errors.vi"("error in (no error)"=w64, "specific error code to clear (0: all)"=1) -> ("error out"=w63:errorcluster)  [unwired: 4 in, 1 out]
          }
          event Panel Close? {
            w68 = TRUE  # Discard the event, the MHL is responsible for closing and stopping this VI.
            # "Hide the panel or send the 'Exit' message if the user clicks the 'X' on the module main VI panel."
            n106 = event-data() -> ()  [unwired: 1 in, 1 out]
            n107 = property class="Module Admin"(reference=w66) -> ("Accessors:External Launch"=w65:bool)  [unwired: 1 in, 2 out]
            n108 = case shown="False" w65 {
              tunnel: w67 -> [_ w73]
              tunnel: [_ w74] -> w69
              frame True {
                # "If externally launched, clicking the 'X' hides the panel, but doesn't close it."
                n109 = control-ref of="This VI"() -> (w70:refnum<vi>)
                n110 = call "Hide VI Panel.vi"("VI"=w70) -> ()  [unwired: 10 in, 1 out]
              }
              frame False {
                # "If run as a stand-alone VI, clicking the panel 'X' stops the VI."
                n111 = call-poly <vilib>:"Delacor_lib_QMH_Enqueue Message (poly).vi"("Priority Message? (F)"=TRUE, "Message"="Exit", "Message Queue in"=w73) -> ("error out"=w74:errorcluster)  [unwired: 7 in, 1 out]
              }
            }
            n112 = event-data("Discard?"=w68) -> ()  [unwired: 1 in, 1 out]
          }
          event User Event {
            # "Another Module called the \"Update analysis parameters\" API Method."
            n113 = event-data() -> ("Contact"=w80:T19, "Decimation"=w79:T2, "Savitzksky-Golay"=w78:T20, "Wait Notifier"=w77:refnum<notifier>, "wait for reply"=w76:bool)  [unwired: 1 in]
            n114 = Bundle(cluster=T7 {"Contact"={"Contact stat?"=TRUE, "Contact Spread of dev"=0.0}, "Decimation"={"App"={"Dec"=1, "apply"=FALSE}, "Con"={"Dec"=1, "apply"=FALSE}, "Ret"={"Dec"=1, "apply"=FALSE}}, "Savitzksky-Golay"={"Sidepoints (M)"=20.0, "Filter Order"=5}, "Wait Notifier"=refnum, "wait for reply"=FALSE} ("Update analysis parameters Argument"), "Contact"=w80, "Decimation"=w79, "Savitzksky-Golay"=w78, "Wait Notifier"=w77, "wait for reply"=w76) -> (w81:T7)
            n115 = call-poly <vilib>:"Delacor_lib_QMH_Enqueue Message (poly).vi"("Message Data"=w81, "Message"="Update analysis parameters", "Message Queue in"=w84) -> ("error out"=w75:errorcluster)  [unwired: 7 in, 1 out]
          }
          event User Event {
            # "Another Module called the \"Update Savitzky parameters\" API Method."
            n116 = event-data() -> ("Savitzksky-Golay"=w86:T20)  [unwired: 1 in]
            n117 = Bundle(cluster=T8 {"Savitzksky-Golay"={"Sidepoints (M)"=20.0, "Filter Order"=5}} ("Update Savitzky parameters Argument"), "Savitzksky-Golay"=w86) -> (w87:T8)
            n118 = call-poly <vilib>:"Delacor_lib_QMH_Enqueue Message (poly).vi"("Message Data"=w87, "Message"="Update Savitzky parameters", "Message Queue in"=w90) -> ("error out"=w85:errorcluster)  [unwired: 7 in, 1 out]
          }
          event User Event {
            # "Another Module called the \"Update decimation\" API Method."
            n119 = event-data() -> ("Decimation"=w92:T2)  [unwired: 1 in]
            n120 = Bundle(cluster=T9 {"Decimation"={"App"={"Dec"=1, "apply"=FALSE}, "Con"={"Dec"=1, "apply"=FALSE}, "Ret"={"Dec"=1, "apply"=FALSE}}} ("Update decimation Argument"), "Decimation"=w92) -> (w93:T9)
            n121 = call-poly <vilib>:"Delacor_lib_QMH_Enqueue Message (poly).vi"("Message Data"=w93, "Message"="Update decimation", "Message Queue in"=w96) -> ("error out"=w91:errorcluster)  [unwired: 7 in, 1 out]
          }
          event User Event {
            # "Another Module called the \"Update contact parameters\" API Method."
            n122 = event-data() -> ("Contact"=w98:T19)  [unwired: 1 in]
            n123 = Bundle(cluster=T10 {"Contact"={"Contact stat?"=TRUE, "Contact Spread of dev"=0.0}} ("Update contact parameters Argument"), "Contact"=w98) -> (w99:T10)
            n124 = call-poly <vilib>:"Delacor_lib_QMH_Enqueue Message (poly).vi"("Message Data"=w99, "Message"="Update contact parameters", "Message Queue in"=w102) -> ("error out"=w97:errorcluster)  [unwired: 7 in, 1 out]
          }
          event User Event {
            # "Another Module called the \"Update Tau delay (ms)\" API Method."
            n125 = event-data() -> ("Tau Delay (ms)"=w104:dbl)  [unwired: 1 in]
            n126 = Bundle(cluster=T11 {"Tau Delay (ms)"=0.0} ("Update Tau delay (ms) Argument"), "Tau Delay (ms)"=w104) -> (w105:T11)
            n127 = call-poly <vilib>:"Delacor_lib_QMH_Enqueue Message (poly).vi"("Message Data"=w105, "Message"="Update Tau delay (ms)", "Message Queue in"=w108) -> ("error out"=w103:errorcluster)  [unwired: 7 in, 1 out]
          }
          event User Event {
            # "Another Module called the \"Open Fcurve object\" API Method."
            n128 = event-data() -> ("Group metadata"=w114:T13, "Channel name(s)"=w113:string[], "Channel datum out"=w112:waveform(dbl)[], "Wait Notifier"=w111:refnum<notifier>, "wait for reply"=w110:bool)  [unwired: 1 in]
            n129 = Bundle(cluster=T12 {"Group metadata"={"property names"=[], "property values"=[]}, "Channel name(s)"=[], "Channel datum out"=[], "Wait Notifier"=refnum, "wait for reply"=FALSE} ("Open Fcurve object Argument"), "Group metadata"=w114, "Channel name(s)"=w113, "Channel datum out"=w112, "Wait Notifier"=w111, "wait for reply"=w110) -> (w115:T12)
            n130 = call-poly <vilib>:"Delacor_lib_QMH_Enqueue Message (poly).vi"("Message Data"=w115, "Message"="Open Fcurve object", "Message Queue in"=w118) -> ("error out"=w109:errorcluster)  [unwired: 7 in, 1 out]
          }
        }
        n131 = call-dynamic "Delacor_lib_QMH_Error Handler - Event Handling Loop.vi"("error in"=w38, "Message Queue in"=w32) -> ("dup error in"=w37:errorcluster)  [unwired: 8 in, 1 out]
      }
    }
    frame Error {
      # "Synchronize Caller Events.vi will inform Start Module.vi that the module has launched and will let the code calling Start Module.vi register for broadcasts and would permit the caller receive the broadcast that an error occurred at launch time."
      n132 = call "Synchronize Caller Events.vi"("Singleton Module Admin in"=w306) -> ("error out"=w311:errorcluster)  [unwired: 9 in, 1 out]
      n133 = call-dynamic "Delacor_lib_QMH_Release Message Queue.vi"("error in"=w303, "Message Queue"=w304) -> ("error out"=w302:errorcluster)  [unwired: 9 in]
      n134 = call "Module Name--constant.vi"() -> ("Module Name"=w309:string)  [unwired: 11 in]
      n135 = case "Settings Editor was\nalready running?" shown="False" w305 {
        frame False {
          n136 = call "Module Name--constant.vi"() -> ("Module Name"=w314:string)  [unwired: 11 in]
          n137 = call "Stop Module.vi"("Wait for Module to Stop? (F)"=TRUE, "Origin"=w314) -> ()  [unwired: 9 in, 1 out]
        }
        frame True {
          # "Another Module is\nin charge of stopping Settings Editor"
        }
      }
      n138 = Format Into String(format string="An error occurred during initialization. %s is no longer running.", w309) -> (resulting string=w307:string)  [unwired: 2 in, 1 out]
      n139 = Merge Errors(w302, w311) -> (w312:errorcluster)
      n140 = call "Error Reported.vi"("Additional Information"=w307, "Error"=w312) -> ()  [unwired: 9 in, 1 out]
    }
  }
  n141 = Merge Errors(w20, w22) -> (w19:errorcluster)
  n142 = call "Close Module.vi"("error in (no error)"=w19, "Module Admin in"=w11) -> ("error out"=w12:errorcluster, "External Launch"=w5:bool, "Module Admin out"=w6:refnum<class "Delacor_lib_QMH_Module Admin.lvclass">)  [unwired: 7 in]
  n143 = Unregister For Events(event registration refnum=w10, error in=w12) -> (error out=w18:errorcluster)
  "error out" <- w18
  n144 = case "External Launch?" shown="True" w5 {
    tunnel: w18 -> [_ w315]
    frame False {
    }
    frame True {
      n145 = case shown="No Error" w315 {
        frame No Error {
          n146 = invoke class="VI" method="FP.Close"() -> ()  [unwired: 3 in, 3 out]
        }
        frame Error {
          n147 = invoke class="VI" method="FP.Open"("Activate"=TRUE ("Activate?")) -> ()  [unwired: 4 in, 5 out]
        }
      }
    }
  }
  n148 = local write "Module Admin"(w6) -> ()
